vi "_Main.vi"   [LabVIEW 2017, in "System_Status.lvlib"]
uses:
  System_Status.lvlib
  Competition Code/RoboRio Code/Globals/Global_System_Checks.vi
types:
  T1 = typedef "Control 1.ctl" = cluster{"PDP ":bool, "PCM":bool, "RIO":bool}
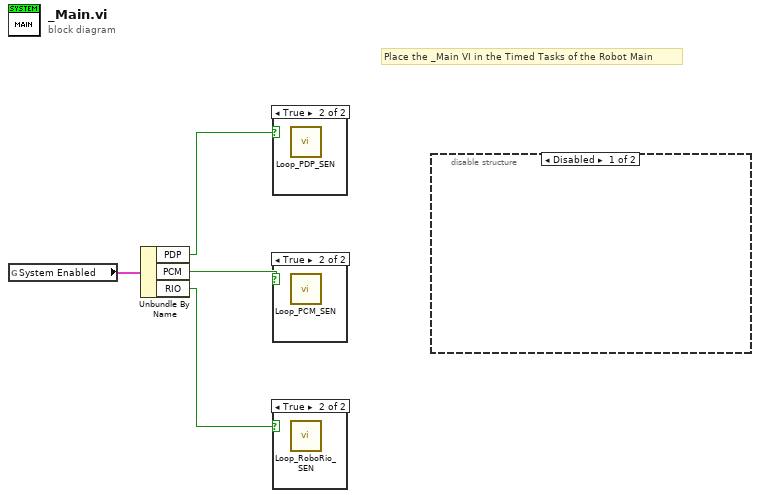
[diagram p0: block diagram]
diagram:
  # "Place the _Main VI in the Timed Tasks of the Robot Main"
  n1 = global read "Global_System_Checks.vi" "System Enabled"() -> (w4:T1)
  n2 = Unbundle By Name(w4) -> ("PDP"=w3:bool, "PCM"=w2:bool, "RIO"=w1:bool)
  n3 = case shown="True" w3 {
    frame False {
    }
    frame True {
      n4 = call "Loop_PDP_SEN.vi"() -> ()  [unwired: 12 in]
    }
  }
  n5 = case shown="True" w2 {
    frame False {
    }
    frame True {
      n6 = call "Loop_PCM_SEN.vi"() -> ()  [unwired: 12 in]
    }
  }
  n7 = case shown="True" w1 {
    frame False {
    }
    frame True {
      n8 = call "Loop_RoboRio_SEN.vi"() -> ()  [unwired: 12 in]
    }
  }
  n9 = disable-structure shown="Disabled" {
    frame Disabled {
    }
    frame Enabled {
    }
  }
